vi "GridView Property Setup.vi"(8 "error in (no error)":errorcluster, 11 ".NET Refnum in":refnum<k24>) -> (0 "error out":errorcluster, 3 ".NET Refnum out":refnum<k24>)   [LabVIEW 2016, in "DataGrid.lvlib" / "DataGridView.lvclass"]
doc: "Sets properties that are not exposed for public inputs as accessors in the class"
uses:
  <userlib>/LabVIEWdotNetDataGrid/source/DataGridView/DataGridView.lvclass
  System.Windows.Forms
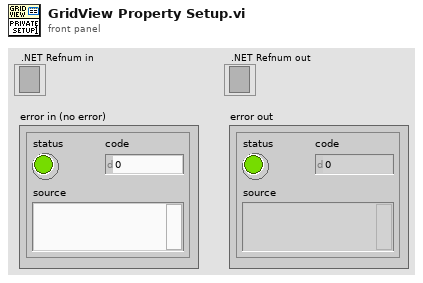
[diagram p1: front panel]
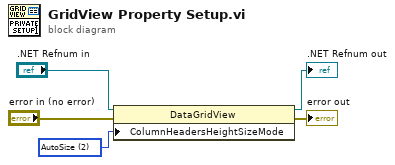
[diagram p0: block diagram]
diagram:
  w2 = 2 items=["EnableResizing", "DisableResizing", "AutoSize"] ("ColumnHeadersHeightSizeMode")
  n1 = property class="DataGridView"(reference=".NET Refnum in", error in="error in (no error)", "ColumnHeadersHeightSizeMode"=w2) -> (reference out=→".NET Refnum out":refnum<k24>, error out=→"error out":errorcluster)
